vi "UpdateStatus.vi"(8 "error in (no error)":errorcluster, 10 "Description":string="Logging Finish!", 11 "Microscope in":refnum<class "Microscope.lvclass">) -> (0 "error out":errorcluster, 3 "Microscope out":refnum<class "Microscope.lvclass">)   [LabVIEW 2020, in "Microscope.lvlib" / "Microscope.lvclass"]
uses:
  Microscope.lvclass
  C:/Program Files/National Instruments/LabVIEW 2020/vi.lib/ActorFramework/Actor/Actor.lvclass
  Component/Device/Device/DataExchange.ctl
  <vilib>/ActorFramework/Actor/Actor.lvclass/Actor.ctl
  Interface/DataListener Messages/OnDataChange Msg/OnDataChange Msg.lvclass/OnDataChange Msg.ctl
  <vilib>/ActorFramework/Message Enqueuer/Message Enqueuer.lvclass/Message Enqueuer.ctl
  <vilib>/ActorFramework/Message Enqueuer/Enqueue.vi
  Interface/DataListener Messages/OnDataChange Msg/OnDataChange Msg.lvclass
  C:/Program Files/National Instruments/LabVIEW 2020/vi.lib/ActorFramework/Message/Message.lvclass
  <vilib>/ActorFramework/Message Priority Queue/Priority Enqueue.vi
  Interface/DataListener/DataListener.lvclass
  <vilib>/ActorFramework/Actor/Actor.lvclass
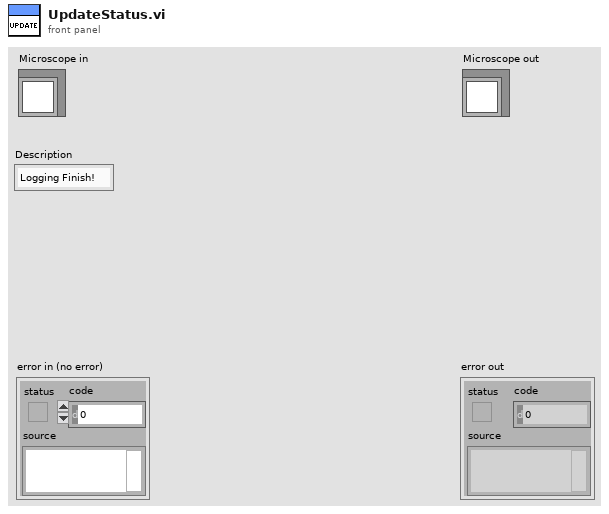
[diagram p1: front panel]
types:
  T1 = typedef "DataListener.lvclass/DataExchange.ctl" = cluster{"Source":string, "Destination":string, "Description":string, "value":variant}
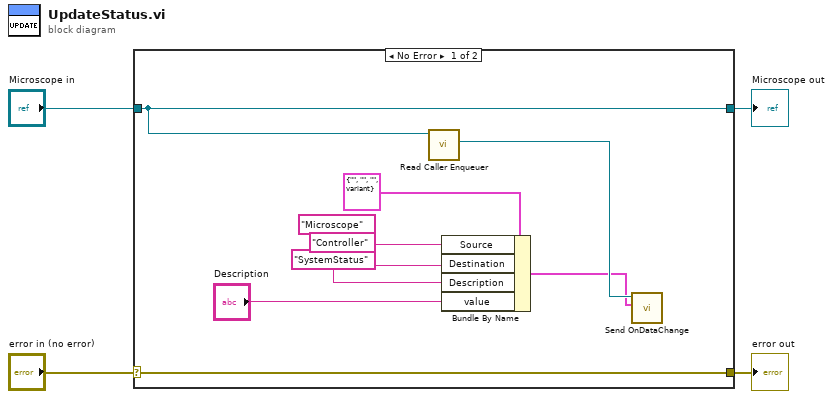
[diagram p0: block diagram]
diagram:
  n1 = case shown="No Error" "error in (no error)" {
    selector: "error in (no error)" -> [w5 w15]
    tunnel: [w5 w15] -> w3
    tunnel: [w6 w14] -> w1
    tunnel: "Microscope in" -> [w6 w14]
    frame No Error {
      n2 = call <vilib>:"Read Caller Enqueuer.vi"("Actor"=w6) -> ("Caller Enqueuer"=w8:refnum<class "Message Enqueuer.lvclass">)  [unwired: 10 in]
      n3 = Bundle By Name(cluster=T1 {"Source"="", "Destination"="", "Description"="", "value"=variant} ("DataExchange"), "Source"="Microscope", "Destination"="Controller", "Description"="SystemStatus", "value"="Description") -> (w7:T1)
      n4 = call "Send OnDataChange.vi"("DataExchange"=w7, "Message Enqueuer"=w8) -> ()  [unwired: 8 in, 2 out]
    }
    frame Error {
    }
  }
  "error out" <- w3
  "Microscope out" <- w1
